vi "ShowPlots.vi"(0 "Display State In":T1, 5 "Plot Names":string[](array[string]), 9 "Container State":T2, 11 "error in (no error)":errorcluster) -> (4 "Display State Out":T1, 15 "error out":errorcluster)   [LabVIEW 2014, in "XListGraph.lvlib" / "XListGraph.xctl"]
uses:
  XListGraph.xctl
  <vilib>/_xctls/Container State.ctl
  Ability/State.ctl
  Support/def-XListGraphOper.ctl
  <vilib>/_xctls/XControlSupport.lvlib
panel:
  # "Add Controls & Indicators that form the parameters of the method here. Hook them to the connector pane. Do not delete the controls & indicators that are already hooked to the connector pane.\n \nTo setup the parameters  for this method, right click on this item in the Project Tree & select \"Configure Method...\"."
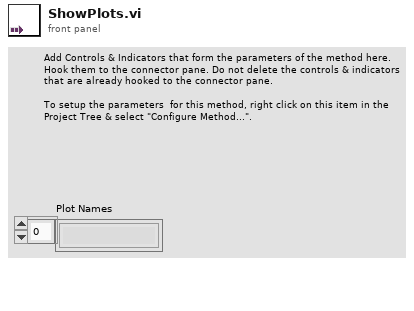
[diagram p1: front panel]
types:
  T1 = typedef "XListGraph.lvlib/XListGraph.xctl/State.ctl" = cluster{"ListWindowSpliterPos":i32, "axes":cluster{"X":cluster{"Label":string, "Unit":string}, "Y":cluster{"Label":string, "Unit":string}}, "Next State":string, "User Event":refnum<user-event>, "Plot Names":string[], "Visible Plot Names":string[], "Selected Plot Names":string[]}
  T2 = typedef "XControlSupport.lvlib/Container State.ctl" = cluster{"Indicator?":bool, "Run Mode?":bool, " Refnum":refnum<vi>}
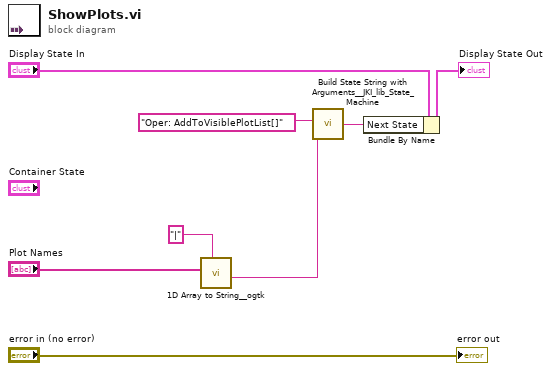
[diagram p0: block diagram]
diagram:
  n1 = call <userlib>:"1D Array to String__ogtk.vi"("delimiter (Tab)"="|", "Array of Strings"="Plot Names") -> ("delimited string"=w1:string)  [unwired: 9 in]
  n2 = call <vilib>:"Build State String with Arguments__JKI_lib_State_Machine.vi"("Arguments (\"\")"=w1, "State"="Oper: AddToVisiblePlotList[]" ("Next State")) -> ("State with Arguments"=w5:string)  [unwired: 4 in]
  n3 = Bundle By Name(cluster="Display State In", "Next State"=w5) -> (→"Display State Out":T1)
  "error out" <- "error in (no error)"
